vi "speed direction.vi"(7 "kp":dbl, 8 "v":dbl, 9 "theta":dbl, 10 "delta y":dbl, 11 "delta x":dbl) -> (3 "newV":dbl)   [LabVIEW 2016]
panel:
  out "angle diff":dbl
  out "alpha":dbl
  out "x-y*floor(x/y)":dbl
  out "y":dbl
  out "x":dbl
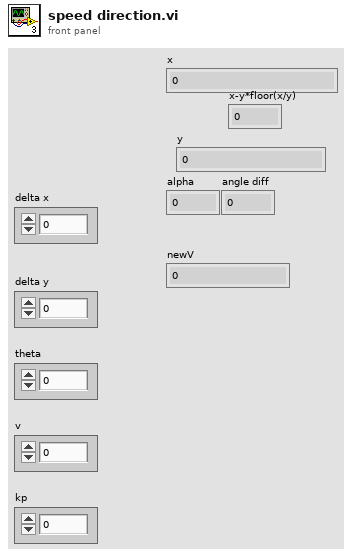
[diagram p1: front panel]
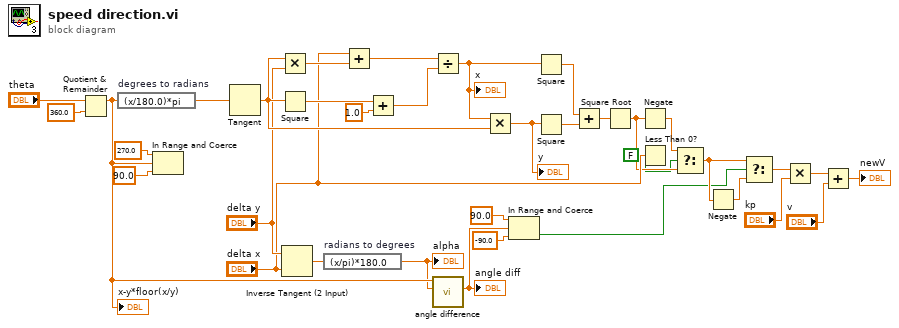
[diagram p0: block diagram]
diagram:
  n1 = Quotient & Remainder(x="theta", y=360.0) -> (x-y*floor(x/y)=w13:dbl)  [unwired: 1 out]
  "x-y*floor(x/y)" <- w13
  n2 = expression code="(x/180.0)*pi" "degrees to radians"(w13) -> (w35:dbl)
  n3 = In Range and Coerce(upper limit=270.0, x=w13, lower limit=90.0) -> ()  [unwired: 2 out]
  n4 = Tangent(1:w35) -> (0:w29:dbl)
  n5 = Multiply(x=w29, y="delta y") -> (x*y=w34:dbl)
  n6 = Square(x=w29) -> (x^2=w33:dbl)
  n7 = Inverse Tangent (2 Input)(1:"delta x", 2:"delta y") -> (0:w14:dbl)
  n8 = expression code="(x/pi)*180.0" "radians to degrees"(w14) -> (w12:dbl)
  "alpha" <- w12
  n9 = Add(x="delta x", y=w34) -> (x+y=w31:dbl)
  n10 = Add(x=w33, y=1.0) -> (x+y=w30:dbl)
  n11 = Divide(x=w31, y=w30) -> (x/y=w24:dbl)
  "x" <- w24
  n12 = call "angle difference.vi"("angle2"=w12, "angle1"=w13) -> ("angle diff"=w8:dbl)  [unwired: 9 in]
  "angle diff" <- w8
  n13 = Multiply(x=w24, y=w29) -> (x*y=w28:dbl)
  "y" <- w28
  n14 = In Range and Coerce(upper limit=90.0, x=w8, lower limit=-90.0) -> (In Range?=w1:bool)  [unwired: 1 out]
  n15 = Square(x=w24) -> (x^2=w26:dbl)
  n16 = Square(x=w28) -> (x^2=w27:dbl)
  n17 = Add(x=w26, y=w27) -> (x+y=w25:dbl)
  n18 = Square Root(x=w25) -> (sqrt(x)=w4:dbl)
  n19 = Negate(x=w4) -> (-x=w5:dbl)
  n20 = Less Than 0?(x="delta x") -> ()  [unwired: 1 out]
  n21 = Select(t=w5, s=FALSE ("x < 0?"), f=w4) -> (s? t:f=w3:dbl)
  n22 = Negate(x=w3) -> (-x=w11:dbl)
  n23 = Select(t=w3, s=w1, f=w11) -> (s? t:f=w22:dbl)
  n24 = Multiply(x=w22, y="kp") -> (x*y=w7:dbl)
  n25 = Add(x=w7, y="v") -> (x+y=→"newV":dbl)
